vi "target_detection.vi"() -> ()   [LabVIEW 2016, in "main.lvrbt"]
uses:
  main.lvrbt
panel:
  out "発見？":bool
  out "距離":dbl
  out "角度":dbl
  out "タイムアウト":bool
  in  "最小部区間幅最大閾値":i32
  in  "最小部区間幅最小閾値":i32
  out "最小部区間下限":i32
  out "最小部区間上限":i32
  out "対象物に差し掛かっている":bool
  out "x >= y?":bool[](array[boolean])
  in  "傾き閾値":i32
  out "配列":dbl[](array[numeric])
  out "dist":dbl
  out "angle":dbl
  in  "sonar_data":dbl[][](array[numeric])
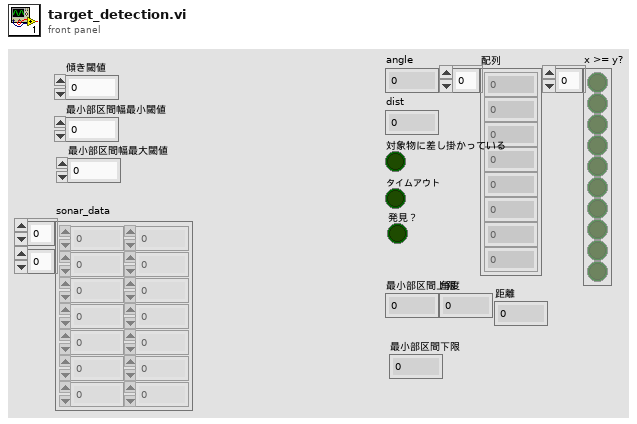
[diagram p1: front panel]
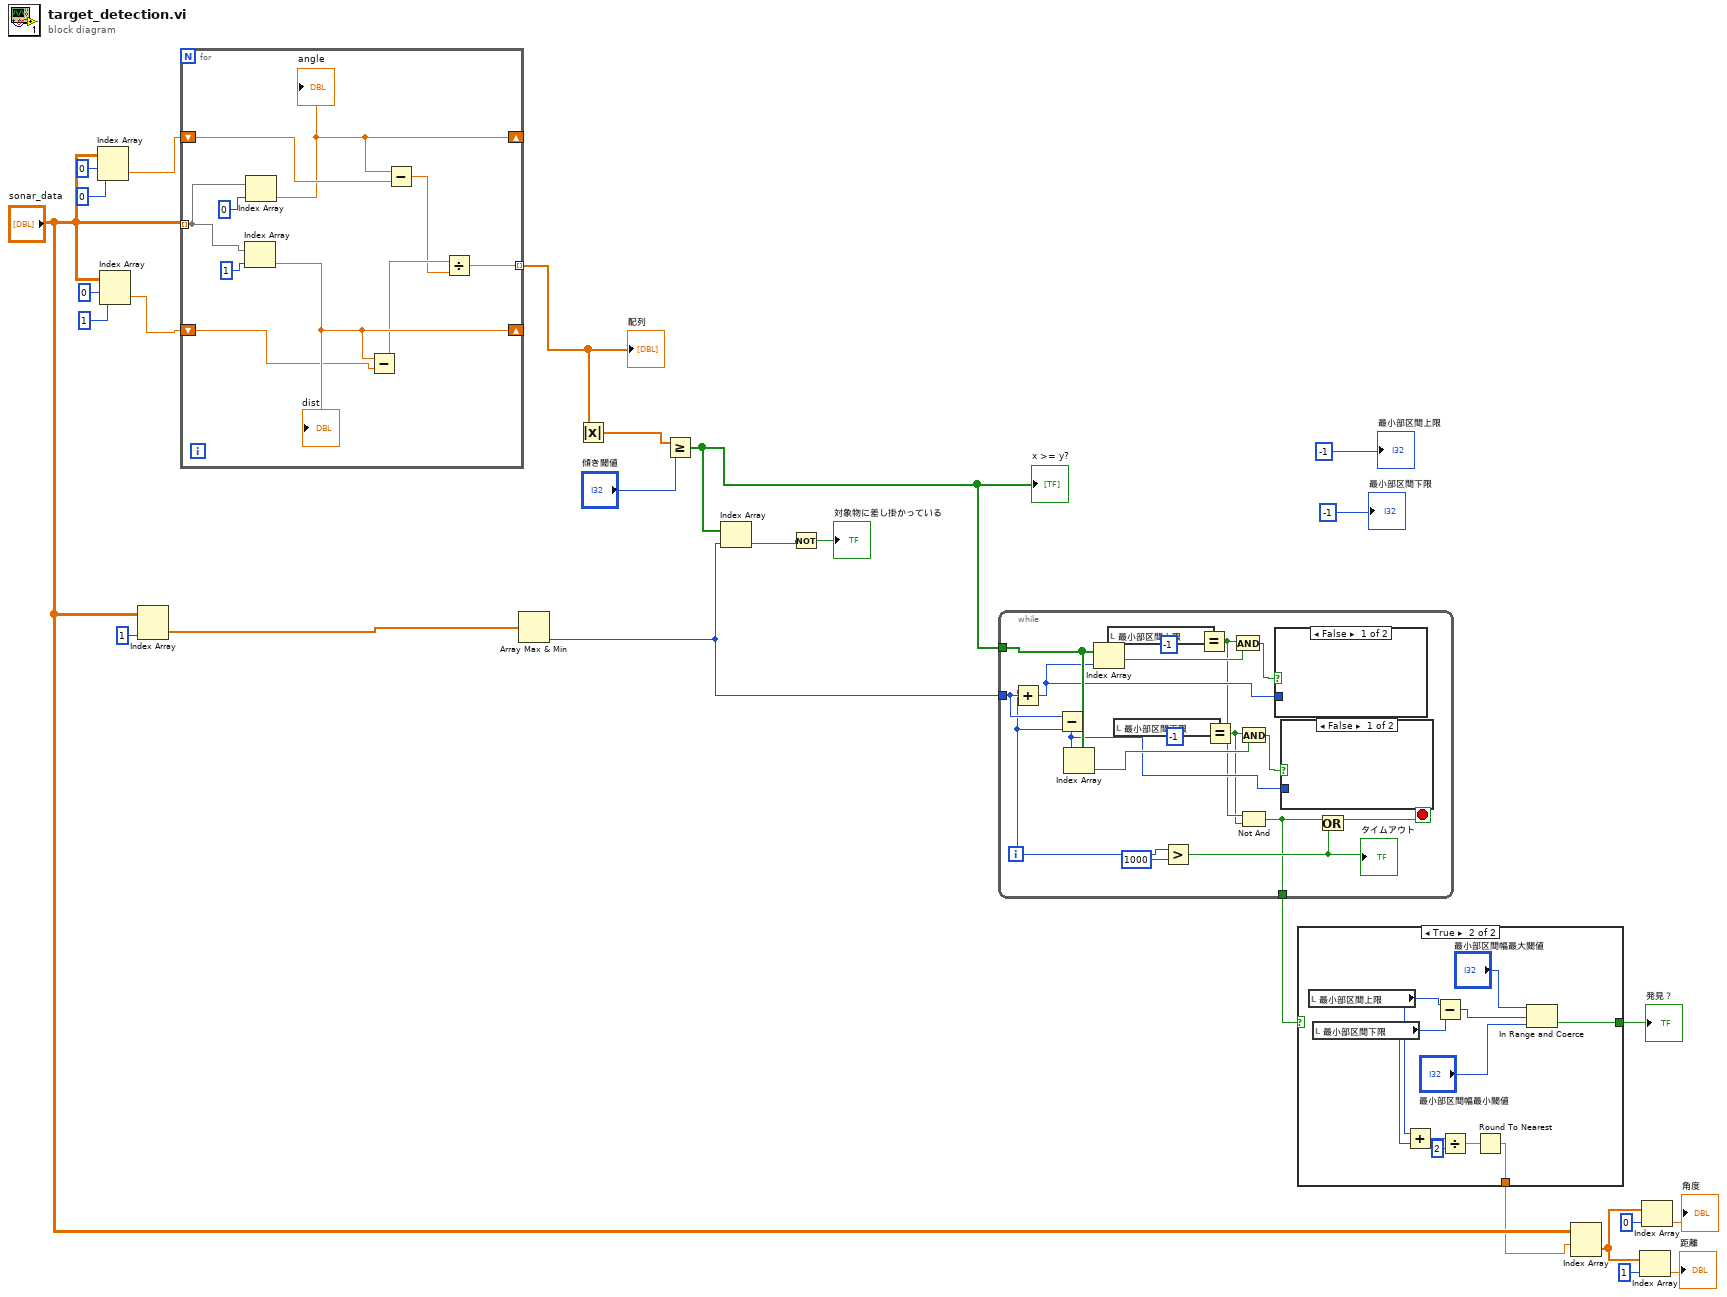
[diagram p0: block diagram]
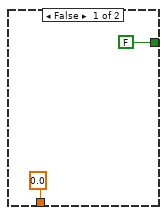
[diagram p2: hidden frame]
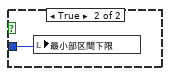
[diagram p3: hidden frame]
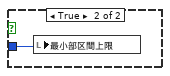
[diagram p4: hidden frame]
diagram:
  n1 = Index Array(array="sonar_data", index (row)=0 ("指標 （行）"), index (col)=0 ("無効な指標 （列）")) -> (element=w22:dbl)
  n2 = Index Array(array="sonar_data", index (row)=0 ("指標 （行）"), index (col)=1 ("無効な指標 （列）")) -> (element=w21:dbl)
  n3 = Index Array(array="sonar_data", index (col)=1 ("無効な指標 （列）")) -> (element=w17:dbl[])  [unwired: 1 in]
  n4 = for {
    tunnel: "sonar_data" -> [w36] mode=indexing
    shift-right: [w32] -> _
    shift-left: w22 -> [w33]
    shift-right: [w31] -> _
    shift-left: w21 -> [w30]
    tunnel: [w27] -> w20 mode=indexing
    n5 = Index Array(array=w36, index=1) -> (element=w31:dbl)
    "dist" <- w31
    n6 = Index Array(array=w36, index=0) -> (element=w32:dbl)
    "angle" <- w32
    n7 = Subtract(x=w31, y=w30) -> (x-y=w29:dbl)
    n8 = Subtract(x=w32, y=w33) -> (x-y=w28:dbl)
    n9 = Divide(x=w29, y=w28) -> (x/y=w27:dbl)
  }
  "配列" <- w20
  n10 = Array Max & Min(array=w17) -> (min index (indices)=w12:i32)  [unwired: 3 out]
  n11 = Absolute Value(x=w20) -> (abs(x)=w19:dbl[])
  n12 = Greater Or Equal?(x=w19, y="傾き閾値") -> (x >= y?=w13:bool[])
  "x >= y?" <- w13
  n13 = Index Array(array=w13, index=w12) -> (element=w15:bool)
  n14 = Not(x=w15) -> (.not. x?=→"対象物に差し掛かっている":bool)
  n15 = while {
    tunnel: w13 -> [w54]
    tunnel: w12 -> [w55]
    tunnel: [w37] -> w9
    i -> [w41]
    stop <- w39 stop-if-true
    n16 = Add(x=w41, y=w55) -> (x+y=w49:i32)
    n17 = Subtract(x=w55, y=w41) -> (x-y=w44:i32)
    n18 = Index Array(array=w54, index=w44) -> (element=w45:bool)
    n19 = Index Array(array=w54, index=w49) -> (element=w53:bool)
    n20 = local read "最小部区間上限"() -> (w52:i32)
    n21 = local read "最小部区間下限"() -> (w46:i32)
    n22 = Greater?(x=w41, y=1000) -> (0:w38:bool)
    "タイムアウト" <- w38
    n23 = Equal?(x=w52, y=-1) -> (x = y?=w43:bool)
    n24 = Equal?(x=w46, y=-1) -> (x = y?=w42:bool)
    n25 = And(x=w43, y=w53) -> (x .and. y?=w50:bool)
    n26 = And(x=w42, y=w45) -> (x .and. y?=w48:bool)
    n27 = Not And(1:w42, 2:w43) -> (0:w37:bool)
    n28 = case shown="FALSE" w50 {
      tunnel: w49 -> [_ w57]
      frame False {
      }
      frame True {
        n29 = local write "最小部区間上限"(w57) -> ()
      }
    }
    n30 = case shown="FALSE" w48 {
      tunnel: w44 -> [_ w56]
      frame False {
      }
      frame True {
        n31 = local write "最小部区間下限"(w56) -> ()
      }
    }
    n32 = Or(x=w37, y=w38) -> (x .or. y?=w39:bool)
  }
  n33 = case shown="TRUE" w9 {
    tunnel: [0.0 w61] -> w7
    tunnel: [FALSE w60] -> w1
    frame False {
    }
    frame True {
      n34 = local read "最小部区間上限"() -> (w66:i32)
      n35 = local read "最小部区間下限"() -> (w65:i32)
      n36 = Add(x=w66, y=w65) -> (x+y=w64:i32)
      n37 = Subtract(x=w66, y=w65) -> (x-y=w68:i32)
      n38 = Divide(x=w64, y=2) -> (x/y=w62:dbl)
      n39 = Round To Nearest(number=w62) -> (nearest integer value=w61:dbl)
      n40 = In Range and Coerce(upper limit="最小部区間幅最大閾値", x=w68, lower limit="最小部区間幅最小閾値") -> (In Range?=w60:bool)  [unwired: 1 out]
    }
  }
  "発見？" <- w1
  n41 = Index Array(array="sonar_data", index (row)=w7) -> (element=w6:dbl[])  [unwired: 1 in]
  n42 = Index Array(array=w6, index=1 ("指標")) -> (element=→"距離":dbl)
  n43 = Index Array(array=w6, index=0 ("指標")) -> (element=→"角度":dbl)
  "最小部区間上限" <- -1
  "最小部区間下限" <- -1
